vi "Get Command strings.vi"() -> ()   [LabVIEW 2022 SP3]
panel:
  out "subarray":string[][](array[string])
  in  "Path":path=path "C:/EnFlo Software MATLAB/input/1D/Data/Titles.txt"
  out "All":string[](array[string])=["pFigureNr", "fAxisLabelX", "fAxisLabelY", "fAxisLabelYrightZloc", "fTitle", "fAxisLimX", "fAxisLimY", "fAxisLimYrightZloc", "fLogAxis", "fInterpreterText", "fShowFigure", "fFigRenderer", "fGrid", "fGridMinor", "fTickLabel", "fFontSize", "fShowLegend", "fShowLegendBox", "fLegendLocation", "fLegendTitle", "fErrorbarOrientation", "fErrorbarColumn", "fYrightAxisColor", "pAxisYright", "pLegendLabel", "pLineColor", "pLineStyle", "pLineWidth", "pLineMarker", "pMarkerSize", "pFitOn", "pFitIndepAxis", "pFitEquation", "pFitStart", "pFitLowerBound", "pFitUpperBound", "pFitIndepAxisFitRange", "pFitIndepAxisPlotRange", "sSavePlot", "sFormatFig", "sLeftEdge", "sBottomEdge", "sPlotHeight", "sPlotWidth", "lLocationAct", "lListFiguresShown", "lLocationFilename", "lLocationTranslations", "lLocationRotations", "lFaceColor", "lEdgeColor", "lFaceTransparency", "lEdgeTransparency", "lViewAngles", "lRefPointCoord", "lRefPointColor", "lRefPointSize", "lRefArrowBaseCoord", "lRefArrowComponents", "lRefArrowColor", "lRefArrowSize", "mPlotAct", "mFormatFig", "mResolution", "mMainTitle", "mGraphsxColumn", "mGraphsxRow", "mLeftEdge", "mRightEdge", "mTopEdge", "mBottomEdge", "mSpaceX", "mSpaceY", "mPlotHeight", "mPlotWidth", "mMainTitleFontSize", "mFontSize", "mShowLegendBox", "mLegendTitle", "mInterpreterText", "mFigRenderer", "mLegendLocation", "mLegendColumnNr"]
  in  "length":i32=100
  in  "index":i32=1
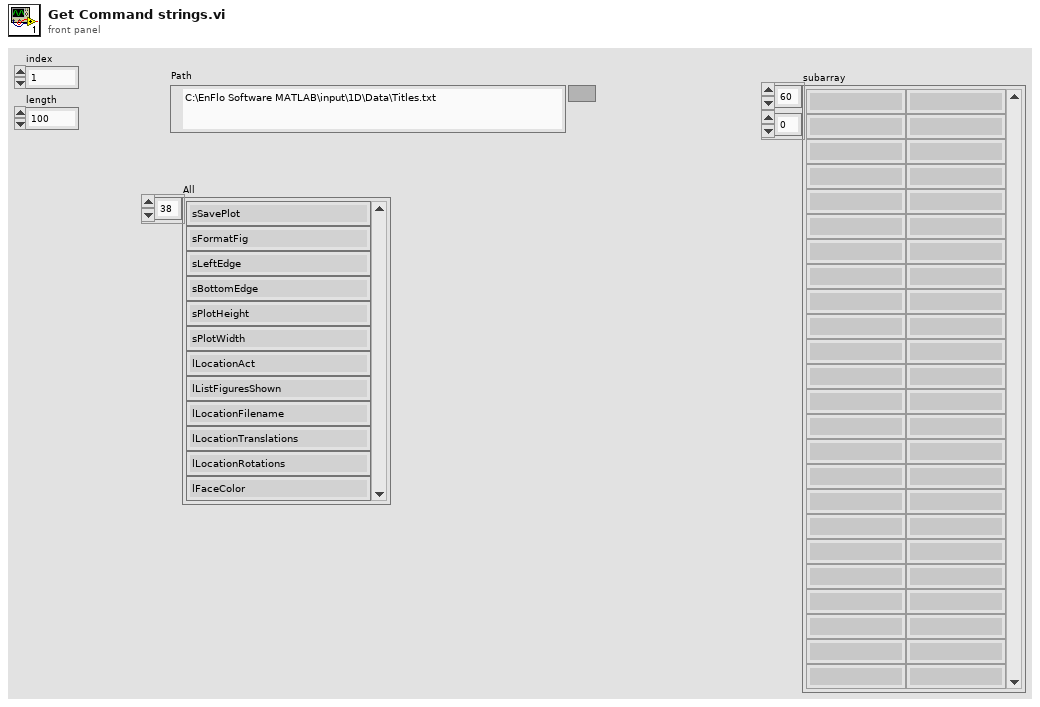
[diagram p1: front panel]
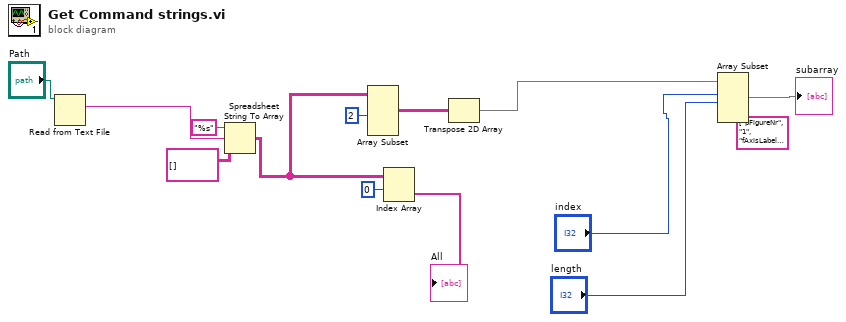
[diagram p0: block diagram]
diagram:
  (unwired) string[][] [["pFigureNr", "1"], ["fAxisLabelX", ""], ["fAxisLabelY", "$z\\ \\mathrm{(mm)}$"], ["fAxisLabelYrightZloc", ""], ["fTitle", "$\\overline{U}/U_{REF}$"], ["fAxisLimX", ""], ["fAxisLimY", ""], ["fAxisLimYrightZloc", ""], ["fLogAxis", "0;0;0"], ["fInterpreterText", "latex"], ["fShowFigure", "0"], ["fFigRenderer", "painters"], ["fGrid", "1;0"], ["fGridMinor", "0;0"], ["fTickLabel", "1;1;1"], ["fFontSize", "10"], ["fShowLegend", "1"], ["fShowLegendBox", "1"], ["fLegendLocation", "best"], ["fLegendTitle", "$x\\ \\mathrm{\\left(mm\\right)}$"], ["fErrorbarOrientation", "horizontal"], ["fErrorbarColumn", "1"], ["fYrightAxisColor", ""], ["pAxisYright", "0"], ["pLegendLabel", "12470"], ["pLineColor", "#FF0000"], ["pLineStyle", "-"], ["pLineWidth", "0.5"], ["pLineMarker", "+"], ["pMarkerSize", "4"], ["pFitOn", "1"], ["pFitIndepAxis", "Y"], ["pFitEquation", "0.064/0.4*log((Y - C(1))/C(2))"], ["pFitStart", "[2 3 4 5 6;10 10 10 15 20]"], ["pFitLowerBound", "0;0"], ["pFitUpperBound", "10;70"], ["pFitIndepAxisFitRange", "0;300"], ["pFitIndepAxisPlotRange", "40;1000"], ["sSavePlot", "0"], ["sFormatFig", "png"], ["sLeftEdge", "0.5"], ["sBottomEdge", "4.85"], ["sPlotHeight", "20"], ["sPlotWidth", "20"], ["lLocationAct", "0"], ["lListFiguresShown", ""], ["lLocationFilename", ""], ["lLocationTranslations", ""], ["lLocationRotations", ""], ["lFaceColor", ""], ["lEdgeColor", ""], ["lFaceTransparency", ""], ["lEdgeTransparency", ""], ["lViewAngles", ""], ["lRefPointCoord", ""], ["lRefPointColor", ""], ["lRefPointSize", ""], ["lRefArrowBaseCoord", ""], ["lRefArrowComponents", ""], ["lRefArrowColor", ""], ["lRefArrowSize", ""], ["mPlotAct", "1"], ["mFormatFig", "pdf"], ["mResolution", "r300"], ["mMainTitle", "Fitting features examples"], ["mGraphsxColumn", "2"], ["mGraphsxRow", "2"], ["mLeftEdge", "2"], ["mRightEdge", "0.8"], ["mTopEdge", "1.5"], ["mBottomEdge", "2.5"], ["mSpaceX", "1"], ["mSpaceY", "1.5"], ["mPlotHeight", "21"], ["mPlotWidth", "29.7"], ["mMainTitleFontSize", "12"], ["mFontSize", "10"], ["mShowLegendBox", "0"], ["mLegendTitle", "$x\\ \\mathrm{\\left(mm\\right)}$"], ["mInterpreterText", "latex"], ["mFigRenderer", "painters"], ["mLegendLocation", "0.5;0.05"], ["mLegendColumnNr", "5"]] ("subarray")
  n1 = Read from Text File(file (use dialog)="Path") -> (text=w13:string)  [unwired: 3 in, 3 out]
  n2 = Spreadsheet String To Array(format string="%s", spreadsheet string=w13, array type (2D Dbl)=string[][] []) -> (array=w7:string[][])  [unwired: 1 in]
  n3 = Array Subset(array=w7, length (row)=2 ("length")) -> (w5:string[][])  [unwired: 3 in]
  n4 = Index Array(array=w7, index (row)=0) -> (element=→"All":string[])  [unwired: 1 in]
  n5 = Transpose 2D Array(2D array=w5) -> (transposed array=w2:string[][])
  n6 = Array Subset(array=w2, index (row)="index", length (row)="length") -> (→"subarray":string[][])  [unwired: 2 in]
